vi "Player Info.vi"(11 "Impenetrable In":refnum<class "Impenetrable.lvclass">) -> (0 "Defeat Speech":string, 1 "Victory Speech":string, 2 "Name":string, 3 "Impenetrable Out":refnum<class "Impenetrable.lvclass">)   [LabVIEW 2015, in "Impenetrable.lvclass"]
uses:
  Impenetrable.lvclass
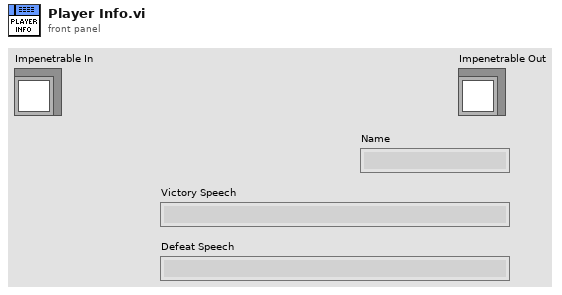
[diagram p1: front panel]
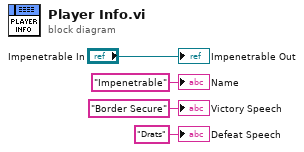
[diagram p0: block diagram]
diagram:
  "Impenetrable Out" <- "Impenetrable In"
  "Name" <- "Impenetrable" ("Name")
  "Victory Speech" <- "Border Secure" ("Victory Speech")
  "Defeat Speech" <- "Drats" ("Defeat Speech")
